vi "Reset.vi"(8 "error in (no error)":errorcluster, 11 "DPO4104 in":refnum<class "DPO4104.lvclass">) -> (0 "error out":errorcluster, 3 "DPO4104 out":refnum<class "DPO4104.lvclass">)   [LabVIEW 2018, in "DPO4104.lvlib" / "DPO4104.lvclass"]
uses:
  DPO4104.lvclass
  PPLs/Oscilloscope/Parent/Oscilloscope.lvlibp/Oscilloscope.lvclass
  <instrlib>/Tektronix DPO MSO 2000 4000 Series/Tektronix DPO MSO 2000 4000 Series.lvlib
  C:/Projects/LabVIEW/PPLs/Oscilloscope/Parent/Oscilloscope.lvlibp/Oscilloscope.lvclass
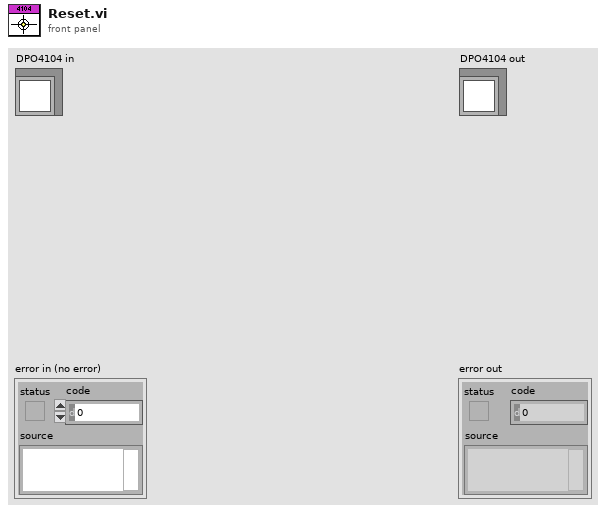
[diagram p1: front panel]
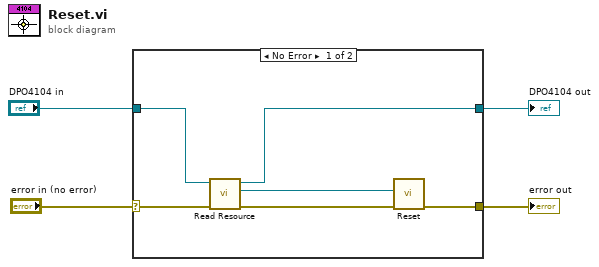
[diagram p0: block diagram]
diagram:
  n1 = case shown="No Error" "error in (no error)" {
    selector: "error in (no error)" -> [w10 w12]
    tunnel: [w6 w12] -> w3
    tunnel: [w8 w11] -> w2
    tunnel: "DPO4104 in" -> [w9 w11]
    frame No Error {
      n2 = call "Read Resource.vi"("error in (no error)"=w10, "Oscilloscope in"=w9) -> ("error out"=w7:errorcluster, "Resource"=w5:refnum<visa-resource-name>, "Oscilloscope out"=w8:refnum<class "DPO4104.lvclass">)  [unwired: 7 in]
      n3 = call <instrlib>:"Reset.vi"("error in (no error)"=w7, "VISA resource name"=w5) -> ("error out"=w6:errorcluster)  [unwired: 8 in, 1 out]
    }
    frame Error {
    }
  }
  "error out" <- w3
  "DPO4104 out" <- w2
